vi "Motion Profile Generater-Optimized.vi"(0 "Max Speed (rotations/sec)":dbl, 5 "Max Acceleration (rotations/sec^2)":dbl, 7 "Max Jerk (rotations/sec^3)":dbl, 9 "Rotations to Travel":dbl, 11 "Motion Profile Control Frame Rate":dbl) -> (4 "Position rotations":dbl[](array[numeric]), 6 "velocity rotations/sec":dbl[](array[numeric]))   [LabVIEW 2015]
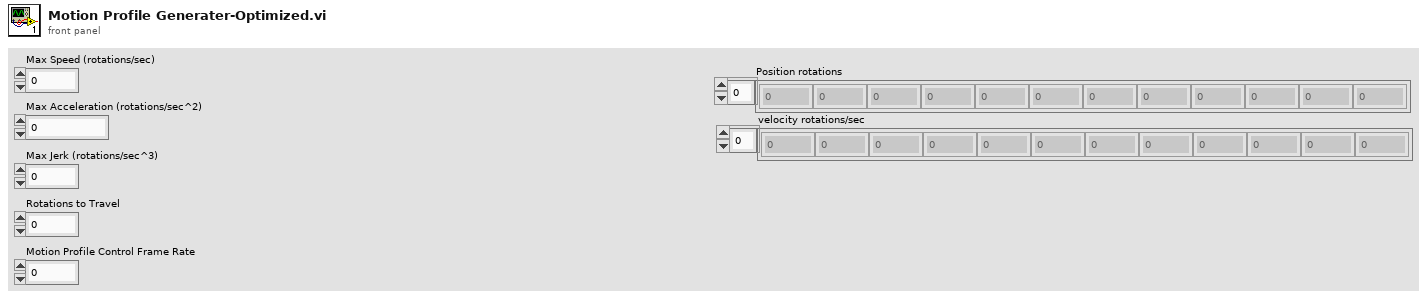
[diagram p1: front panel]
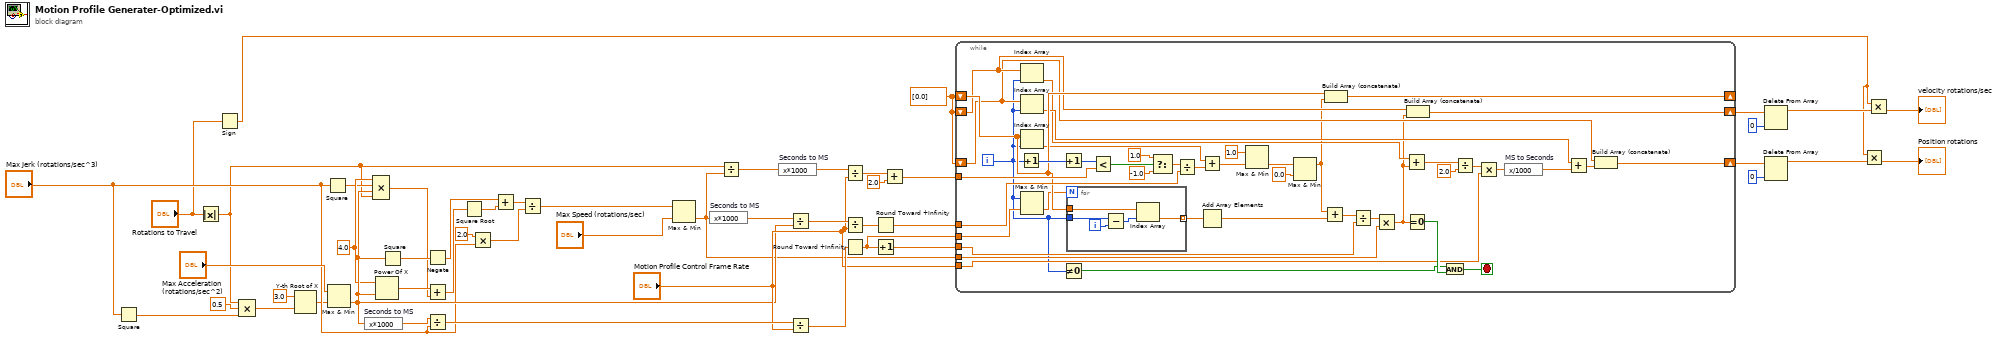
[diagram p0: block diagram]
diagram:
  w29 = dbl[] [0.0] ("Array")
  w20 = 4.0 ("x")
  n1 = Square(x="Max Jerk (rotations/sec^3)") -> (x^2=w26:dbl)
  n2 = Absolute Value(x="Rotations to Travel") -> (abs(x)=w5:dbl)
  n3 = Sign(1:"Rotations to Travel") -> (0:w1:dbl)
  n4 = Compound Arithmetic op=MULTIPLY(w5, 0.5 ("value"), w26) -> (w25:dbl)
  n5 = Y-th Root of X(1:w25, 2:3.0 ("y")) -> (0:w28:dbl)
  n6 = Square(x="Max Jerk (rotations/sec^3)") -> (x^2=w19:dbl)
  n7 = Max & Min(x="Max Acceleration (rotations/sec^2)", y=w28) -> (min(x,y)=w33:dbl)  [unwired: 1 out]
  n8 = expression code="x*1000" "Seconds to MS"(w33) -> (w49:dbl)
  n9 = Compound Arithmetic op=MULTIPLY(w20, w19, w33, w5) -> (w18:dbl)
  n10 = Power Of X(1:w33, 2:w20) -> (0:w21:dbl)
  n11 = Square(x=w33) -> (x^2=w23:dbl)
  n12 = Negate(x=w23) -> (-x=w22:dbl)
  n13 = Add(x=w21, y=w18) -> (x+y=w17:dbl)
  n14 = Divide(x=w49, y="Max Jerk (rotations/sec^3)") -> (x/y=w39:dbl)
  n15 = Square Root(x=w17) -> (sqrt(x)=w15:dbl)
  n16 = Multiply(x=2.0, y="Max Jerk (rotations/sec^3)") -> (x*y=w12:dbl)
  n17 = Add(x=w22, y=w15) -> (x+y=w14:dbl)
  n18 = Divide(x=w14, y=w12) -> (x/y=w13:dbl)
  n19 = Max & Min(x=w13, y="Max Speed (rotations/sec)") -> (min(x,y)=w31:dbl)  [unwired: 1 out]
  n20 = expression code="x*1000" "Seconds to MS"(w31) -> (w48:dbl)
  n21 = Divide(x=w5, y=w31) -> (x/y=w47:dbl)
  n22 = expression code="x*1000" "Seconds to MS"(w47) -> (w46:dbl)
  n23 = Divide(x=w48, y=w33) -> (x/y=w42:dbl)
  n24 = Divide(x=w39, y="Motion Profile Control Frame Rate") -> (x/y=w38:dbl)
  n25 = Divide(x=w46, y="Motion Profile Control Frame Rate") -> (x/y=w45:dbl)
  n26 = Divide(x=w42, y="Motion Profile Control Frame Rate") -> (x/y=w41:dbl)
  n27 = Round Toward +Infinity(x=w38) -> (ceil(x): smallest int >= x=w37:dbl)
  n28 = Round Toward +Infinity(x=w41) -> (ceil(x): smallest int >= x=w40:dbl)
  n29 = Increment(x=w37) -> (x+1=w36:dbl)
  n30 = Add(x=w45, y=2.0) -> (x+y=w43:dbl)
  n31 = while {
    tunnel: w43 -> [w92]
    shift-right: [w79] -> _
    shift-left: w29 -> [w78]
    tunnel: w40 -> [w84]
    tunnel: w37 -> [w76]
    tunnel: w36 -> [w72]
    tunnel: w31 -> [w70]
    shift-right: [w69] -> w7
    shift-left: w29 -> [w67]
    shift-right: [w68] -> w11
    shift-left: w29 -> [w61]
    tunnel: "Motion Profile Control Frame Rate" -> [w51]
    i -> [w50]
    stop <- w54 stop-if-true
    n32 = Increment(x=w50) -> (x+1=w81:i32)
    n33 = Index Array(array=w67, index=w50) -> (element=w58:dbl)
    n34 = Index Array(array=w61, index=w50) -> (element=w60:dbl)
    n35 = Index Array(array=w78, index=w50) -> (element=w52:dbl)
    n36 = Max & Min(x=w50, y=w76) -> (min(x,y)=w75:dbl)  [unwired: 1 out]
    n37 = Increment(x=w81) -> (x+1=w82:i32)
    n38 = Not Equal To 0?(x=w50) -> (x != 0?=w55:bool)
    n39 = for {
      N: w75 -> [_]
      tunnel: w50 -> [w96]
      tunnel: w78 -> [w94]
      tunnel: [w93] -> w77 mode=indexing
      i -> [w97]
      n40 = Subtract(x=w96, y=w97) -> (x-y=w95:i32)
      n41 = Index Array(array=w94, index=w95) -> (element=w93:dbl)
    }
    n42 = Less?(x=w82, y=w92) -> (x < y?=w88:bool)
    n43 = Select(t=1.0, s=w88, f=-1.0) -> (s? t:f=w85:dbl)
    n44 = Divide(x=w85, y=w84) -> (x/y=w83:dbl)
    n45 = Add(x=w52, y=w83) -> (x+y=w80:dbl)
    n46 = Add Array Elements(numeric array=w77) -> (sum=w74:dbl)
    n47 = Max & Min(x=1.0, y=w80) -> (min(x,y)=w90:dbl)  [unwired: 1 out]
    n48 = Max & Min(x=w90, y=0.0) -> (max(x,y)=w53:dbl)  [unwired: 1 out]
    n49 = Add(x=w53, y=w74) -> (x+y=w73:dbl)
    n50 = Build Array (concatenate)(w78, w53) -> (w79:dbl[])
    n51 = Divide(x=w73, y=w72) -> (x/y=w71:dbl)
    n52 = Multiply(x=w71, y=w70) -> (x*y=w57:dbl)
    n53 = Add(x=w58, y=w57) -> (x+y=w66:dbl)
    n54 = Equal To 0?(x=w57) -> (x = 0?=w56:bool)
    n55 = Build Array (concatenate)(w67, w57) -> (w69:dbl[])
    n56 = And(x=w55, y=w56) -> (x .and. y?=w54:bool)
    n57 = Divide(x=w66, y=2.0) -> (x/y=w64:dbl)
    n58 = Multiply(x=w64, y=w51) -> (x*y=w63:dbl)
    n59 = expression code="x/1000" "MS to Seconds"(w63) -> (w62:dbl)
    n60 = Add(x=w60, y=w62) -> (x+y=w59:dbl)
    n61 = Build Array (concatenate)(w61, w59) -> (w68:dbl[])
  }
  n62 = Delete From Array(array=w7, index=0) -> (array with subset deleted=w6:dbl[])  [unwired: 1 in, 1 out]
  n63 = Delete From Array(array=w11, index=0) -> (array with subset deleted=w9:dbl[])  [unwired: 1 in, 1 out]
  n64 = Multiply(x=w1, y=w9) -> (x*y=→"Position rotations":dbl[])
  n65 = Multiply(x=w1, y=w6) -> (x*y=→"velocity rotations/sec":dbl[])
